vi "UEGO card.vi"(8 "error in (no error)":errorcluster, 11 "Node Ptr":T3 format="%.0x") -> (0 "error out":errorcluster)   [LabVIEW 2014, in "SLSC configuration System Explorer.lvlib"]
uses:
  SLSC configuration System Explorer.lvlib
  <vilib>/NI Veristand/Custom Device API/Custom Device Item Ref.ctl
  Type Defs/Card Position.ctl
  Shared/SPI Utility/Slot #.ctl
  Shared/Constants.vi
  <vilib>/NI Veristand/Custom Device API/Get Item Property (U32).vi
  <vilib>/NI Veristand/Custom Device API/Get Item Property (String).vi
  <vilib>/NI Veristand/Custom Device API/Set Item Property (U32).vi
  <vilib>/NI Veristand/Custom Device API/Custom Device API.lvlib
  Shared/SLSC configuration Shared.lvlib
panel:
  out "FPGA Item Name":string
  in  "Header 3":cluster{"Section Name":string}={"Section Name"="Oxygen Sensor Simulation Card Settings"}
  in  "Header 2":cluster{"Section Name":string}={"Section Name"="Oxygen Sensor Simulation Card Settings"}
  in  "Calibration Time (µsec)":u32
  in  "Hardware Settling Time (µsec)":u32
  in  "Card Position":T1 {"Slot #" max=15}
  in  "Header":cluster{"Section Name":string}={"Section Name"="Oxygen Sensor Simulation Card Settings"}
  in  "Description":string
  in  "Name":string
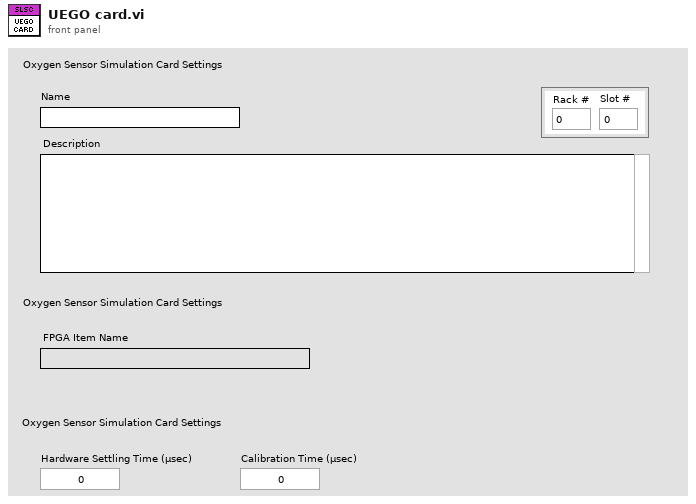
[diagram p1: front panel]
types:
  T1 = typedef "SLSC configuration Shared.lvlib/Card Position.ctl" = cluster{"Rack #":u8, "Slot #":T2}
  T2 = typedef "SLSC configuration Shared.lvlib/Slot #.ctl" = u8
  T3 = typedef "Custom Device API.lvlib/Custom Device Item Ref.ctl" = u64
  T4 = typedef "Custom Device API.lvlib/Custom Device Commands.ctl" = enum16{"Default", "Item renamed", "Shutdown", "Dynamic button pressed"}
  T5 = typedef "Custom Device API.lvlib/Custom Device Item Info.ctl" = cluster{"Name":string, "Is Channel":bool, "GUID":string, "Is Waveform":bool}
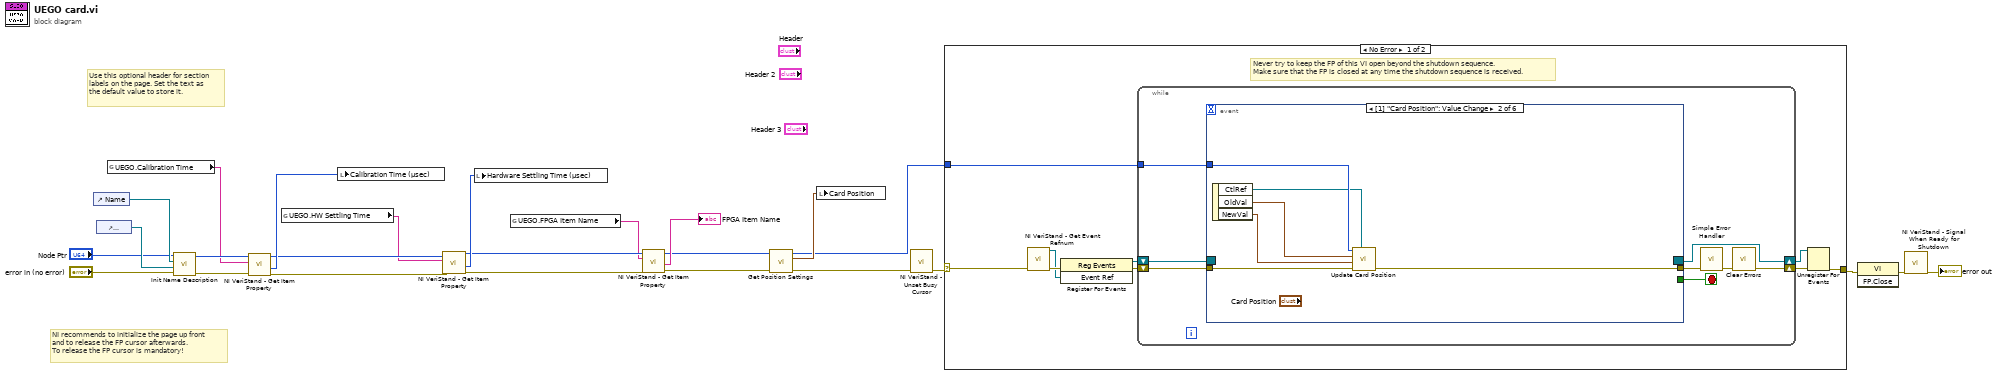
[diagram p0: block diagram]
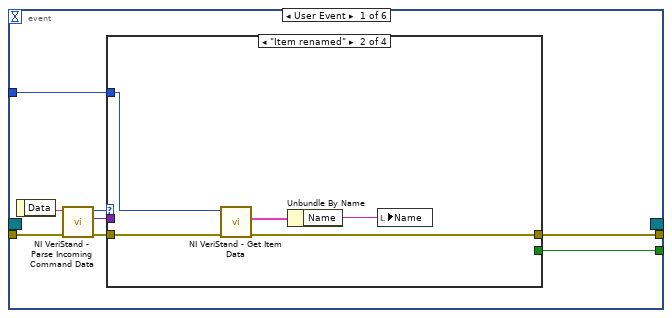
[diagram p2: hidden frame]
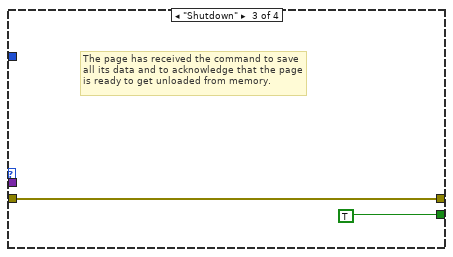
[diagram p4: hidden frame]
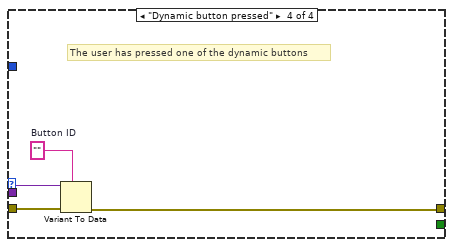
[diagram p5: hidden frame]
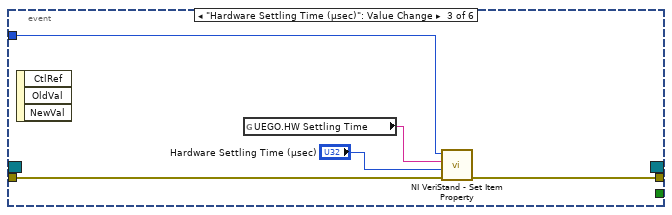
[diagram p6: hidden frame]
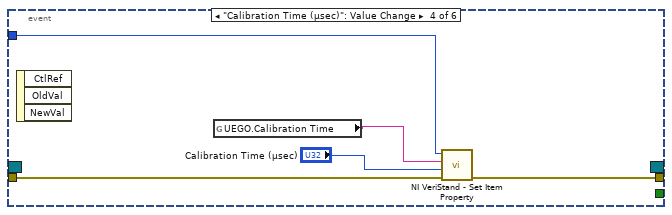
[diagram p7: hidden frame]
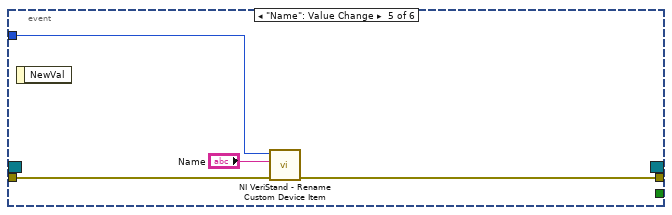
[diagram p8: hidden frame]
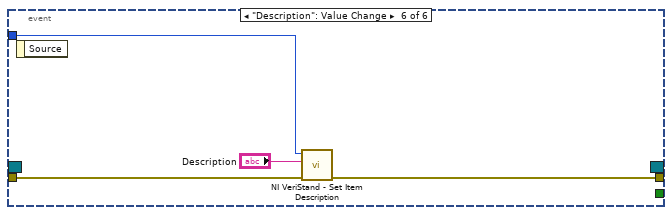
[diagram p9: hidden frame]
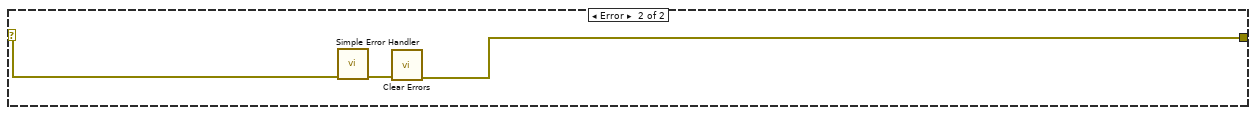
[diagram p10: hidden frame]
diagram:
  # "Use this optional header for section labels on the page. Set the text as the default value to store it."
  # "NI recommends to initialize the page up front\nand to release the FP cursor afterwards.\nTo release the FP cursor is mandatory!"
  n1 = control-ref of="Name"() -> (w21:refnum<vi>)
  n2 = control-ref of="Description"() -> (w20:refnum<vi>)
  n3 = global read "Constants.vi" "UEGO.Calibration Time"() -> (w12:string)
  n4 = call "Init Name Description.vi"("error in (no error)"="error in (no error)", "Description"=w20, "Name"=w21, "Node Ptr"="Node Ptr") -> ("error out"=w14:errorcluster, "Node Ptr out"=w13:T3)  [unwired: 6 in]
  n5 = call-poly <vilib>:"NI VeriStand - Get Item Property.vi"("error in (no error)"=w14, "Property Name"=w12, "Item Ref in"=w13) -> ("error out"=w10:errorcluster, "Value"=w11:u32, "Item Ref out"=w9:T3)  [unwired: 5 in, 1 out]
  n6 = global read "Constants.vi" "UEGO.HW Settling Time"() -> (w8:string)
  n7 = local write "Calibration Time (µsec)"(w11) -> ()
  n8 = call-poly <vilib>:"NI VeriStand - Get Item Property.vi"("error in (no error)"=w10, "Property Name"=w8, "Item Ref in"=w9) -> ("error out"=w6:errorcluster, "Value"=w7:u32, "Item Ref out"=w5:T3)  [unwired: 5 in, 1 out]
  n9 = local write "Hardware Settling Time (µsec)"(w7) -> ()
  n10 = global read "Constants.vi" "UEGO.FPGA Item Name"() -> (w4:string)
  n11 = call-poly <vilib>:"NI VeriStand - Get Item Property.vi"("error in (no error)"=w6, "Property Name"=w4, "Item Ref in"=w5) -> ("error out"=w1:errorcluster, "Value"=→"FPGA Item Name":string, "Item Ref out"=w2:T3)  [unwired: 5 in, 1 out]
  n12 = call "Get Position Settings.vi"("error in (no error)"=w1, "Item Ref in"=w2) -> ("error out"=w16:errorcluster, "Card Position"=w17:T1, "Item Ref out"=w15:T3)  [unwired: 7 in]
  n13 = local write "Card Position"(w17) -> ()
  n14 = call <vilib>:"NI VeriStand - Unset Busy Cursor.vi"("error in (no error)"=w16) -> ("error out"=w22:errorcluster)  [unwired: 10 out]
  n15 = case shown="No Error" w22 {
    selector: w22 -> [w27 w89]
    tunnel: [w31 w87] -> w25
    tunnel: w15 -> [w26 _]
    frame No Error {
      # "Never try to keep the FP of this VI open beyond the shutdown sequence.\nMake sure that the FP is closed at any time the shutdown sequence is received."
      n16 = call <vilib>:"NI VeriStand - Get Event Refnum.vi"("error in (no error)"=w27) -> ("error out"=w34:errorcluster, "Event Ref"=w30:refnum<user-event>)  [unwired: 9 out]
      n17 = register-events(error in=w34, w30) -> (reference out=w28:refnum<event-registration>, error out=w29:errorcluster)  [unwired: 1 in]
      n18 = while {
        shift-right: [w36] -> w32
        shift-left: w29 -> [w41]
        shift-right: [w42] -> w33
        shift-left: w28 -> [w40]
        tunnel: w26 -> [w35]
        stop <- w39 stop-if-true
        n19 = event shown="[1] \"Card Position\": Value Change" {
          selector: w40 -> [_ _ _ _ _ _]
          dyn-events: [_ _ _ _ _ _] -> w42
          timeout: _ -> [_ _ _ _ _ _]
          tunnel: w41 -> [w50 w68 w73 w78 w82 w86]
          tunnel: [w46 _ _ _ _ _] -> w39
          tunnel: [w45 w63 w72 w77 w81 w85] -> w38
          tunnel: w35 -> [w43 w65 w70 w76 w79 w83]
          event User Event {
            n20 = event-data() -> ("Data"=w49:string)  [unwired: 1 out]
            n21 = call <vilib>:"NI VeriStand - Parse Incoming Command Data.vi"("error in (no error)"=w50, "Incoming data"=w49) -> ("error out"=w48:errorcluster, "Outgoing data"=w44:variant, "Action"=w47:T4)  [unwired: 7 out]
            n22 = case shown="\"Item renamed\"" w47 {
              tunnel: w48 -> [w51 w56 w57 w62]
              tunnel: [_ _ TRUE _] -> w46
              tunnel: [w51 w54 w57 w59] -> w45
              tunnel: w44 -> [_ _ _ w61]
              tunnel: w43 -> [_ w52 _ _]
              frame "Default", Default {
              }
              frame "Item renamed" {
                n23 = call <vilib>:"NI VeriStand - Get Item Data.vi"("error in (no error)"=w56, "Item Ref in"=w52) -> ("error out"=w54:errorcluster, "Item Info"=w55:T5)  [unwired: 8 out]
                n24 = Unbundle By Name(w55) -> ("Name"=w53:string)
                n25 = local write "Name"(w53) -> ()
              }
              frame "Shutdown" {
                # "The page has received the command to save all its data and to acknowledge that the page is ready to get unloaded from memory."
              }
              frame "Dynamic button pressed" {
                w60 = ""  # Button ID
                # "The user has pressed one of the dynamic buttons"
                n26 = Variant To Data(error in=w62, type=w60, Variant=w61) -> (error out=w59:errorcluster)  [unwired: 1 out]
              }
            }
          }
          event Value Change {
            n27 = event-data() -> ("CtlRef"=w64:refnum<vi>, "OldVal"=w66:T1, "NewVal"=w67:T1)  [unwired: 1 out]
            n28 = call "Update Card Position.vi"("Card Position Ref"=w64, "error in (no error)"=w68, "NewVal"=w67, "OldVal"=w66, "Node Ptr in"=w65) -> ("error out"=w63:errorcluster)  [unwired: 6 in]
          }
          event "Hardware Settling Time (µsec)": Value Change {
            n29 = event-data() -> ()  [unwired: 4 out]
            n30 = global read "Constants.vi" "UEGO.HW Settling Time"() -> (w69:string)
            n31 = call-poly <vilib>:"NI VeriStand - Set Item Property.vi"("error in (no error)"=w73, "Value"="Hardware Settling Time (µsec)", "Property Name"=w69, "Item Ref in"=w70) -> ("error out"=w72:errorcluster)  [unwired: 5 in, 2 out]
          }
          event "Calibration Time (µsec)": Value Change {
            n32 = event-data() -> ()  [unwired: 4 out]
            n33 = global read "Constants.vi" "UEGO.Calibration Time"() -> (w74:string)
            n34 = call-poly <vilib>:"NI VeriStand - Set Item Property.vi"("error in (no error)"=w78, "Value"="Calibration Time (µsec)", "Property Name"=w74, "Item Ref in"=w76) -> ("error out"=w77:errorcluster)  [unwired: 5 in, 2 out]
          }
          event "Name": Value Change {
            n35 = event-data() -> ()  [unwired: 2 out]
            n36 = call <vilib>:"NI VeriStand - Rename Custom Device Item.vi"("error in (no error)"=w82, "New Name"="Name", "Item Ref in"=w79) -> ("error out"=w81:errorcluster)  [unwired: 1 in, 7 out]
          }
          event "Description": Value Change {
            n37 = event-data() -> ()  [unwired: 2 out]
            n38 = call <vilib>:"NI VeriStand - Set Item Description.vi"("error in (no error)"=w86, "Description"="Description", "Item Ref in"=w83) -> ("error out"=w85:errorcluster)  [unwired: 8 out]
          }
        }
        n39 = call <vilib>:"Simple Error Handler.vi"("error in (no error)"=w38) -> ("error out"=w37:errorcluster)  [unwired: 1 in, 7 out]
        n40 = call <vilib>:"Clear Errors.vi"("error in (no error)"=w37) -> ("error out"=w36:errorcluster)  [unwired: 1 in, 5 out]
      }
      n41 = Unregister For Events(event registration refnum=w33, error in=w32) -> (error out=w31:errorcluster)
    }
    frame Error {
      n42 = call <vilib>:"Simple Error Handler.vi"("error in (no error)"=w89) -> ("error out"=w88:errorcluster)  [unwired: 1 in, 7 out]
      n43 = call <vilib>:"Clear Errors.vi"("error in (no error)"=w88) -> ("error out"=w87:errorcluster)  [unwired: 1 in, 5 out]
    }
  }
  n44 = invoke class="VI" method="FP.Close"(error in=w25) -> (error out=w24:errorcluster)  [unwired: 2 in, 2 out]
  n45 = call <vilib>:"NI VeriStand - Signal When Ready for Shutdown.vi"("error in (no error)"=w24) -> ("error out"=→"error out":errorcluster)  [unwired: 10 out]
